vi "Check if good target.vi"(6 "Avg Factor":i32, 8 "y2-R":dbl, 9 "x2-R":dbl, 10 "y1-L":dbl, 11 "x1-L":dbl) -> (0 "y2 (R) out":dbl, 1 "x2 (L) out":dbl, 2 "y1 (L) out":dbl, 3 "x1 (L) out":dbl, 5 "Good target?":bool)   [LabVIEW 2018]
uses:
  <vilib>/ptbypt/NI_PtbyPt.lvlib
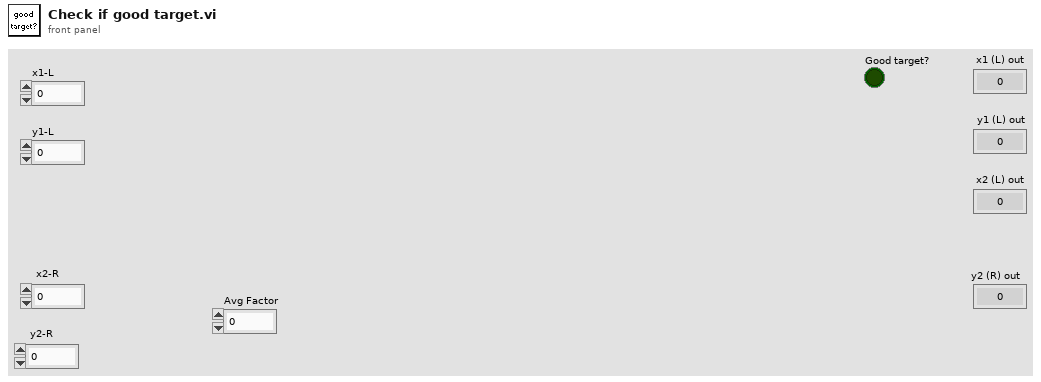
[diagram p1: front panel]
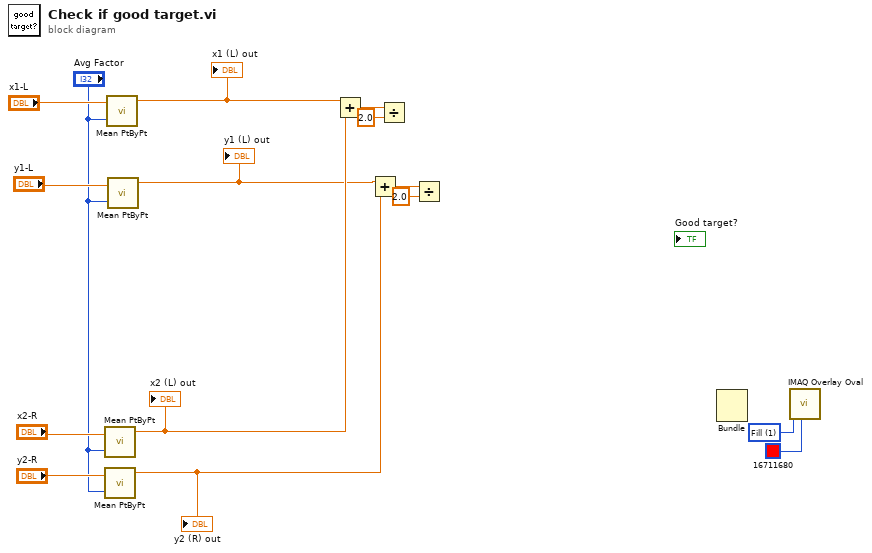
[diagram p0: block diagram]
diagram:
  w10 = u32 1 items=["Frame", "Fill"] ("Drawing Mode (Frame)")
  n1 = call <vilib>:"Mean PtByPt.vi"("x"="x2-R", "sample length"="Avg Factor") -> ("mean"=w7:dbl)  [unwired: 2 in, 1 out]
  "x2 (L) out" <- w7
  n2 = call <vilib>:"Mean PtByPt.vi"("x"="y2-R", "sample length"="Avg Factor") -> ("mean"=w1:dbl)  [unwired: 2 in, 1 out]
  "y2 (R) out" <- w1
  n3 = call <vilib>:"Mean PtByPt.vi"("x"="x1-L", "sample length"="Avg Factor") -> ("mean"=w8:dbl)  [unwired: 2 in, 1 out]
  "x1 (L) out" <- w8
  n4 = call <vilib>:"Mean PtByPt.vi"("x"="y1-L", "sample length"="Avg Factor") -> ("mean"=w2:dbl)  [unwired: 2 in, 1 out]
  "y1 (L) out" <- w2
  n5 = Add(x=w8, y=w7) -> (x+y=w6:dbl)
  n6 = Add(x=w2, y=w1) -> (x+y=w3:dbl)
  n7 = Divide(x=w6, y=2.0) -> ()  [unwired: 1 out]
  n8 = Divide(x=w3, y=2.0) -> ()  [unwired: 1 out]
  n9 = Bundle() -> ()  [unwired: 5 in, 1 out]
  n10 = call "IMAQ Overlay Oval"("Color"=u32 16711680, "Drawing Mode (Frame)"=w10) -> ()  [unwired: 8 in, 2 out]
